vi "Save.vi"(8 "error in (no error)":errorcluster, 11 "Default contorls manipulator in":refnum<class "Default contorls manipulator.lvclass">) -> (0 "error out":errorcluster, 1 "Config path":path caption="Configuration file path (leave empty to load default path)", 2 "VI path":path caption="VI path to load default controls", 3 "Default contorls manipulator out":refnum<class "Default contorls manipulator.lvclass">)   [LabVIEW 2020, in "Default contorls manipulator.lvclass"]
doc: "You do not have to wire anything once the loader run. The internal operation will take over all the stuff.\nNote that the SAVE operation is typically run in the last stage of a program."
uses:
  Default contorls manipulator.lvclass
  Default contorls manipulator.lvclass/Default contorls manipulator.ctl
  Save-Load-Defaults.lvlib/Save-Load-Defaults.lvlib
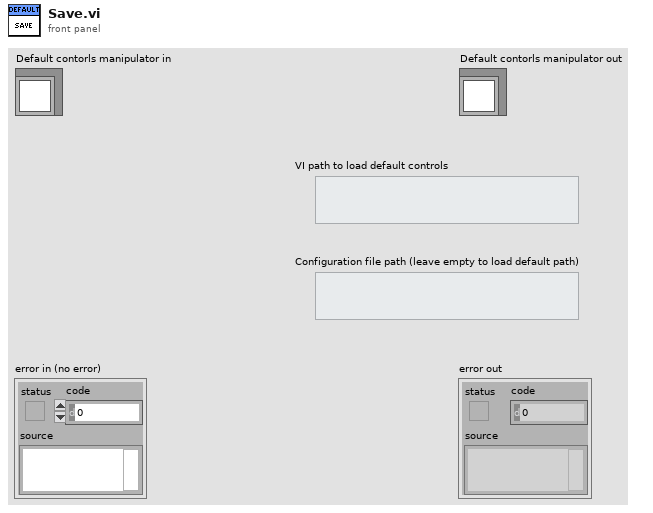
[diagram p1: front panel]
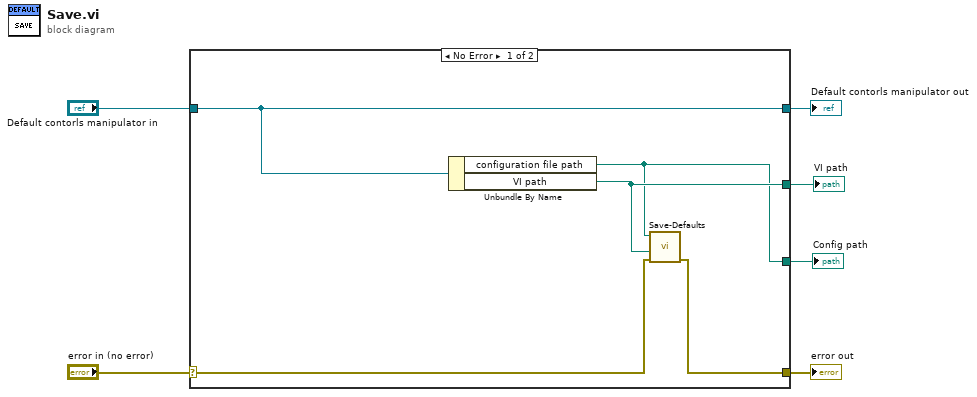
[diagram p0: block diagram]
diagram:
  n1 = case shown="No Error" "error in (no error)" {
    selector: "error in (no error)" -> [w10 w13]
    tunnel: [w9 w13] -> w5
    tunnel: [w11 w12] -> w3
    tunnel: "Default contorls manipulator in" -> [w11 w12]
    tunnel: [w8 _] -> w2
    tunnel: [w7 _] -> w1
    frame No Error {
      n2 = Unbundle By Name(w11) -> ("configuration file path"=w7:path, "VI path"=w8:path)
      n3 = call "Save-Defaults.vi"("error in (no error)"=w10, "VI path"=w8, "configuration file path"=w7) -> ("error out"=w9:errorcluster)  [unwired: 8 in]
    }
    frame Error {
    }
  }
  "error out" <- w5
  "Default contorls manipulator out" <- w3
  "VI path" <- w2
  "Config path" <- w1
